vi "Stimulus-Plot.vi"(0 "AO Control":T1[](xcontrol), 1 "Waveform Graph":refnum<vi>, 5 "Array":dbl[][](array[numeric]), 9 "Sampling Rate (Hz)":dbl, 11 "error in (no error)":errorcluster) -> (4 "AO Control out":T1[](xcontrol), 6 "Array out":dbl[][](array[numeric]), 15 "error out":errorcluster)   [LabVIEW 2020]
doc: "Helper function to plot stimuli in a sensible fashion."
uses:
  Controls/Multichannel XCtl/Multichannel XCtl.xctl
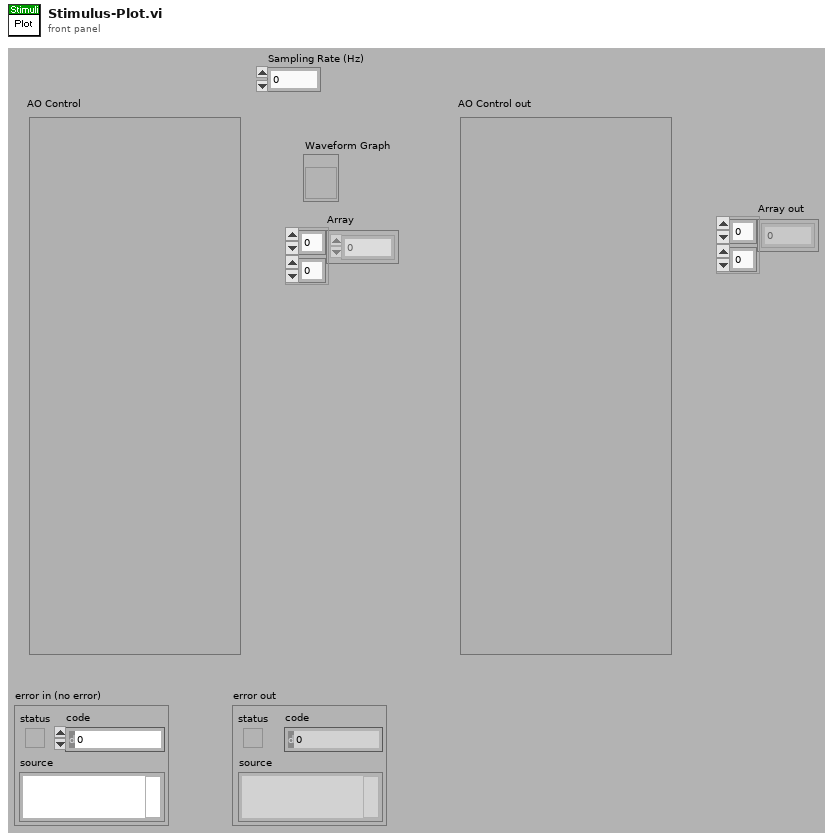
[diagram p1: front panel]
types:
  T1 = typedef "Stimulus Channel.xctl/Stimulus Channel Data.ctl" = cluster{"Waveform":T2, "Filter":T19, "Gate":T20, "Level":T21}
  T2 = typedef "Waveform XCtl.xctl/Waveform Data.ctl" = cluster{"Type":T3, "Tone":T4, "Pulse Train":T5, "Noise":T8, "File":T9, "FMSweep":T10, "Chirp Train":T11, "Complex Tone":cluster{"Params":T13, "Data":T15}, "Moving Ripple":T16}
  T3 = typedef "Waveform Enum.ctl" = enum16{"OFF", "Tone", "Noise", "Pulse Train", "File", "FM Sweep", "Chirp Train", "Complex Tone", "FM Tone", "Moving Ripple"}
  T4 = typedef "Tone Params.ctl" = cluster{"Frequency (kHz)":dbl, "Last Freq":dbl, "Last Phase":dbl}
  T5 = typedef "Pulse Train Params.ctl" = cluster{"Pulse width (us)":dbl, "Pulse rate (Hz)":dbl, "Gap (ms)":dbl, "Polarity":T6, "PT State":T7, "Asynch":bool}
  T6 = typedef "Pulse Polarity.ctl" = enum16{"POS", "NEG", "POS-NEG", "NEG-POS"}
  T7 = typedef "PT-Continuous State.ctl" = cluster{"Template":dbl[], "Nperiod":i32, "Index":i32, "Pulse Rate (Hz)":dbl, "Phase (cycles)":dbl, "Noff":i32}
  T8 = typedef "Noise Params.ctl" = cluster{"InvFilt":bool, "Noise":dbl[], "CurPt":i32, "Aweight":bool, "Seed":i32, "afile":path}
  T9 = typedef "StimFile-Params.ctl" = cluster{"Filename":path, "Signal":dbl[], "Channel":i32, "stream":bool, "offset":i32, "nreps":i32, "loops":i32, "Tokens":i32, "Randomize":bool, "order":i32[]}
  T10 = typedef "FM Sweep Params.ctl" = cluster{"Rate (oct/s)":dbl, "Fmin (Hz)":dbl, "Fmax (Hz)":dbl, "Ramp (ms)":dbl, "Linear":bool}
  T11 = typedef "Chirp Train.ctl" = cluster{"Params":T12, "Data":cluster{"WF":dbl[]}}
  T12 = typedef "Chirp Train Params.ctl" = cluster{"Fmin (kHz)":dbl, "Fmax (kHz)":dbl, "Compensate":bool, "Duration (ms)":dbl}
  T13 = typedef "CT-Params.ctl" = cluster{"F0 (Hz)":dbl, "Band":cluster{"Flow (Hz)":dbl, "Fhigh (Hz)":dbl}, "Phase":T14, "Min F0 (Hz)":dbl, "Max F0 (Hz)":dbl, "ContinRandPhase":bool, "Max peak factor":dbl, "Max mod depth":dbl, "MinHarmNum":i32, "MaxHarmNum":i32, "Level Mode":enum16{"per component", "overall rms"}, "% jitter":dbl}
  T14 = typedef "CT-Phase Enum.ctl" = enum16{"Cosine", "Random", "Alternating"}
  T15 = typedef "CT-Runtime Data.ctl" = cluster{"Ncomp":i32, "MinHarm":i32, "Phase":dbl[], "Amplitude":dbl[], "Npts/frame":i32, "Last F0":dbl, "Fmin":dbl, "Fmax":dbl, "Lslope":dbl, "randphase":bool, "overall rms":bool, "fmult":dbl[], "jittered":bool}
  T16 = typedef "Moving Ripple.ctl" = cluster{"Params":T17, "Data":T18}
  T17 = typedef "Moving Ripple.Params.ctl" = cluster{"Fmin":dbl, "Fmax":dbl, "Density":dbl, "Velocity":dbl, "Depth":dbl, "Phase":dbl, "Comp/oct":i32}
  T18 = typedef "Moving Ripple.Data.ctl" = cluster{"Freq":dbl[], "A":dbl[], "phase":dbl[], "Phase":dbl}
  T19 = typedef "Filter XCtl.xctl/Filter Data.ctl" = cluster{"CF (kHz)":dbl, "BW (kHz)":dbl, "IIR Filter Cluster":cluster{"filter structure":enum32{"IIR 2nd Order", "IIR 4th Order"}, "Reverse Coefficients":dbl[], "Forward Coefficients":dbl[]}, "Final Filter State":dbl[], "Scale Factor":dbl, "Final Filter State 2":dbl[], "Quadrature":bool, "Type":enum16{"Lowpass", "Highpass", "Bandpass", "Bandstop", "OFF"}}
  T20 = typedef "Gate Control.xctl/Gate Data.ctl" = cluster{"Active":bool, "Delay (ms)":dbl, "Width (ms)":dbl, "Ramp (ms)":dbl}
  T21 = typedef "Level XCtl.xctl/Level Data.ctl" = cluster{"Level":dbl, "Units":T22, "Max":dbl, "Multiplier":dbl, "Cal File":path, "Cal":cluster{"Freq (Hz)":dbl[], "Mag (dB SPL)":dbl[], "Phase (deg)":dbl[]}}
  T22 = typedef "Level Units.ctl" = enum16{"dB atten", "dB SPL", "dB re 1 Vrms", "dB V/Hz½", "mW", "dB HL", "Volts", "dB mW"}
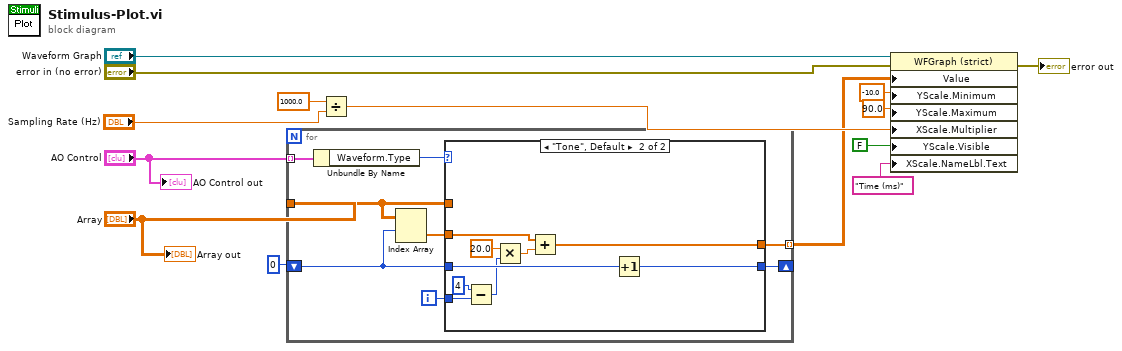
[diagram p0: block diagram]
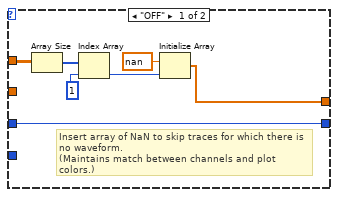
[diagram p2: hidden frame]
diagram:
  n1 = for {
    tunnel: "AO Control" -> [w22] mode=indexing
    shift-right: [w19] -> _
    shift-left: 0 -> [w20]
    tunnel: "Array" -> [w17]
    tunnel: [w15] -> w3 mode=indexing
    i -> [w16]
    n2 = Unbundle By Name(w22) -> ("Waveform.Type"=w21:T3)
    n3 = Index Array(array=w17, index (row)=w20) -> (element=w18:dbl[])  [unwired: 1 in]
    n4 = case shown="\"Tone\", Default" w21 {
      tunnel: w20 -> [w29 w34]
      tunnel: [w29 w38] -> w19
      tunnel: w18 -> [_ w35]
      tunnel: w17 -> [w28 _]
      tunnel: w16 -> [_ w32]
      tunnel: [w23 w30] -> w15
      frame "OFF" {
        # "Insert array of NaN to skip traces for which there is no waveform. \n(Maintains match between channels and plot colors.)"
        n5 = Array Size(array=w28) -> (size(s)=w27:i32[])
        n6 = Index Array(array=w27, index=1) -> (element=w25:i32)
        n7 = Initialize Array(nan ("element"), w25) -> (w23:dbl[])
      }
      frame "Tone", Default {
        n8 = Subtract(x=4, y=w32) -> (x-y=w33:i32)
        n9 = Multiply(x=20.0, y=w33) -> (x*y=w36:dbl)
        n10 = Add(x=w35, y=w36) -> (x+y=w30:dbl[])
        n11 = Increment(x=w34) -> (x+1=w38:i32)
      }
    }
  }
  n12 = Divide(x=1000.0, y="Sampling Rate (Hz)") -> (x/y=w7:dbl)
  n13 = property class="WFGraph (strict)"(reference="Waveform Graph", error in="error in (no error)", "Value"=w3, "YScale.Minimum"=-10.0 ("Y Scale.Range:Minimum"), "YScale.Maximum"=90.0 ("Y Scale.Range:Maximum"), "XScale.Multiplier"=w7, "YScale.Visible"=FALSE ("Y Scale.Name Label.Visible"), "XScale.NameLbl.Text"="Time (ms)" ("X Scale.Name Label.Text")) -> (error out=→"error out":errorcluster)  [unwired: 1 out]
  "AO Control out" <- "AO Control"
  "Array out" <- "Array"
